vi "Lockin.Low Pass Filter (subVI).vi"(8 "error in (no error)":errorcluster, 9 "Element Data":i32, 10 "Array":waveform(dbl)[](array[waveform]), 11 "Lockin.DAQ in":refnum<class "Instrument.DAQ.lvclass">) -> (0 "error out":errorcluster, 1 "Fc (Hz)":dbl, 2 "signal out":waveform(dbl)[](array[waveform]))   [LabVIEW 2019, in "Instrument.DAQ.lvclass"]
uses:
  Instrument.DAQ.lvclass
  Instrument.DAQ.lvclass/Instrument.DAQ.ctl
  <vilib>/addons/Digital Filter Design/Process.llb/DFD Filtering (Array NChan).vi
  <vilib>/addons/Digital Filter Design/Process.llb/DFD Filtering (Wfm NChan).vi
  <vilib>/addons/Digital Filter Design/NI_DigFilterLicensed.lvlib
panel:
  out "Lockin.DAQ out":refnum<class "Instrument.DAQ.lvclass">
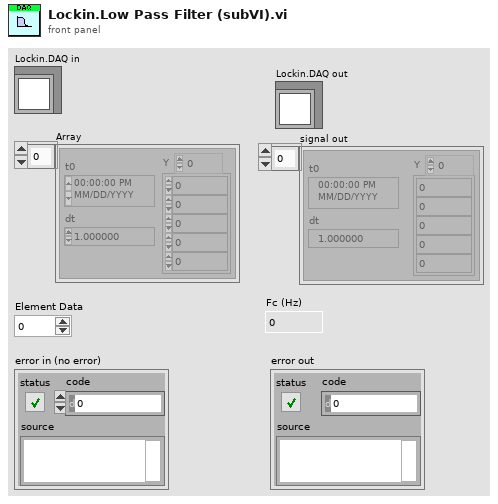
[diagram p1: front panel]
types:
  T1 = typedef "Instrument.DAQ.lvclass/REF.Channel--Cluster--Array.ctl" = T2[]
  T2 = typedef "Instrument.DAQ.lvclass/REF.Channel--Cluster.ctl" = cluster{"Enable?":bool, "Channel":i32, "Frequency":dbl, "Phase":dbl, "TC":dbl, "Roll-Off":i32}
  T3 = enum16{"Lowpass", "Highpass", "Bandpass", "Bandstop"}
  T4 = typedef "NI_DigFilterLicensed.lvlib/DFD Filter Obj.ctl" = cluster{"mSRate_Fs":dbl, "mSRate_Version":string, "mSRate_Comments":string, "mSRate_OrgCoef":T5, "mSRate_CurCoef":T5, "mSRate_Quantized?":bool, "mSRate_QCoef":T5, "mSRate_QSettings":T7[], "mSRate_Order":i32, "mSRate_Scaling":cluster{"mSRate_ScaleByPowerOf2?":bool, "mSRate_ScaleType":T9}}
  T5 = typedef "NI_DigFilterLicensed.lvlib/DFD Filter Coef.ctl" = cluster{"type":T6, "gain":dbl, "coef a (k)":dbl[], "coef b (v)":dbl[]}
  T6 = typedef "NI_DigFilterLicensed.lvlib/DFD Filter Structure Type Selector.ctl" = enum16{"Undefined", "FIR Direct Form", "FIR Direct Form Transposed", "FIR Symmetric", "FIR Antisymmetric", "IIR Direct Form I", "IIR Direct Form I Transposed", "IIR Direct Form II", "IIR Direct Form II Transposed", "IIR Cascaded Second Order Sections Form I", "IIR Cascaded Second Order Sections Form I Transposed", "IIR Cascaded Second Order Sections Form II", "IIR Cascaded Second Order Sections Form II Transposed", "Lattice Allpass (basic sections)", "Lattice Allpass (one multiplier sections)", "Lattice Allpass (normalized sections)", "Lattice AR (basic sections)", "Lattice AR (one multiplier sections)", "Lattice AR (normalized sections)", "Lattice MA (minimum phase)", "Lattice MA (maximum phase)", "Lattice ARMA (basic sections)", "Lattice ARMA (one multiplier sections)", "Lattice ARMA (normalized sections)"}
  T7 = typedef "NI_DigFilterLicensed.lvlib/dfd_Internal Quantization Settings.ctl" = cluster{"source":T8, "wl":i16, "iwl":i16, "overflow mode":enum16{"Saturation", "Wrap"}, "rounding mode":enum16{"Nearest", "Truncation"}, "signed?":bool}
  T8 = typedef "NI_DigFilterLicensed.lvlib/dfd_Internal Quantization Srcs.ctl" = u16
  T9 = typedef "NI_DigFilterLicensed.lvlib/DFD Coef Norm Type.ctl" = enum16{"No Norm", "Time Domain 1-Norm", "Time Domain 2-Norm", "Time Domain Inf-Norm"}
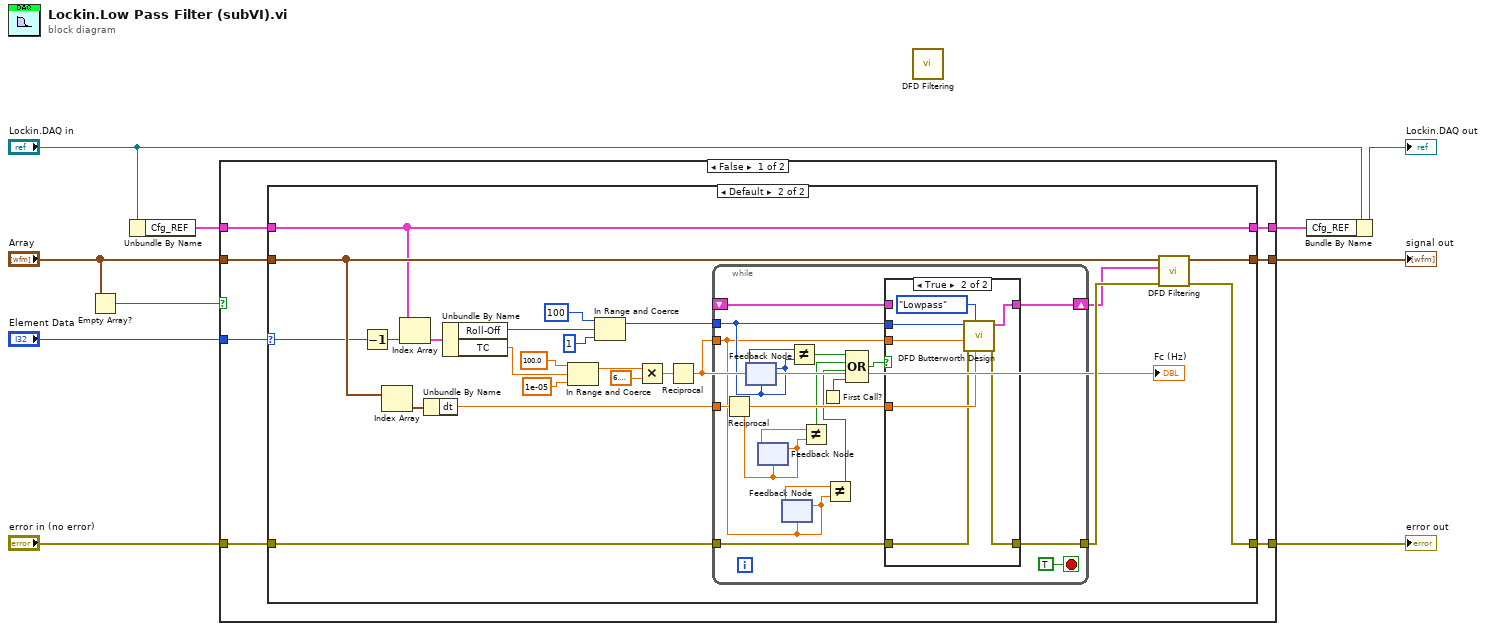
[diagram p0: block diagram]
diagram:
  n1 = Empty Array?(array="Array") -> (empty?=w6:bool)
  n2 = Unbundle By Name("Lockin.DAQ in") -> ("Cfg_REF"=w3:T1)
  n3 = case shown="False" w6 {
    tunnel: "error in (no error)" -> [w17 w72]
    tunnel: [w16 w72] -> w9
    tunnel: [w15 w71] -> w8
    tunnel: "Element Data" -> [w13 _]
    tunnel: "Array" -> [w14 w71]
    tunnel: w3 -> [w12 w70]
    tunnel: [w11 w70] -> w1
    frame False {
      n4 = case shown="Default" w13 {
        selector: w13 -> [_ w26]
        tunnel: w17 -> [w20 w43]
        tunnel: [w20 w22] -> w16
        tunnel: w14 -> [w19 w42]
        tunnel: [w19 w27] -> w15
        tunnel: w12 -> [w18 w21]
        tunnel: [w18 w21] -> w11
        frame 0 {
        }
        frame Default {
          n5 = Decrement(x=w26) -> (x-1=w25:i32)
          n6 = Index Array(array=w42) -> (element=w40:waveform(dbl))  [unwired: 1 in]
          n7 = Index Array(array=w21, index=w25) -> (element=w38:T2)
          n8 = Unbundle By Name(w40) -> ("dt"=w39:dbl)
          n9 = Unbundle By Name(w38) -> ("Roll-Off"=w36:i32, "TC"=w37:dbl)
          n10 = In Range and Coerce(upper limit=100.0, x=w37, lower limit=1e-05) -> (coerced(x)=w29:dbl)  [unwired: 1 out]
          n11 = In Range and Coerce(upper limit=100, x=w36, lower limit=1) -> (coerced(x)=w28:i32)  [unwired: 1 out]
          n12 = Multiply(x=w29, y=6.283185307179586) -> (x*y=w33:dbl)
          n13 = Reciprocal(x=w33) -> (1/x=w24:dbl)
          "Fc (Hz)" <- w24
          n14 = while {
            tunnel: w39 -> [w60]
            tunnel: w28 -> [w55]
            tunnel: w24 -> [w51]
            shift-right: [w46] -> w23
            shift-left: _ -> [w47]
            tunnel: w43 -> [w58]
            tunnel: [w57] -> w41
            stop <- TRUE stop-if-true
            n15 = Reciprocal(x=w60) -> (1/x=w53:dbl)
            n16 = feedback-in #1(w55) -> ()
            n17 = feedback #1(w55) -> (w56:i32)
            n18 = feedback #2(w53) -> (w54:dbl)
            n19 = feedback-in #2(w53) -> ()
            n20 = feedback #3(w51) -> (w52:dbl)
            n21 = feedback-in #3(w51) -> ()
            n22 = Not Equal?(x=w56, y=w55) -> (x != y?=w50:bool)
            n23 = Not Equal?(x=w54, y=w53) -> (x != y?=w49:bool)
            n24 = First Call?() -> (First Call?: T/F=w45:bool)
            n25 = Not Equal?(x=w52, y=w51) -> (x != y?=w48:bool)
            n26 = Compound Arithmetic op=OR(w50, w49, w48, w45) -> (w44:bool)
            n27 = case shown="True" w44 {
              tunnel: w53 -> [_ w69]
              tunnel: w55 -> [_ w67]
              tunnel: w51 -> [_ w66]
              tunnel: w58 -> [w62 w65]
              tunnel: [w62 w64] -> w57
              tunnel: [w61 w63] -> w46
              tunnel: w47 -> [w61 _]
              frame False {
              }
              frame True {
                n28 = call <vilib>:"DFD Butterworth Design.vi"("fs [Hz]"=w69, "filter type"=T3."Lowpass", "error in (no error)"=w65, "low cutoff freq [Hz]"=w66, "order"=w67) -> ("error out"=w64:errorcluster, "filter out"=w63:T4)  [unwired: 5 in]
              }
            }
          }
          n29 = call-poly <vilib>:"DFD Filtering.vi"("error in (no error)"=w41, "filter"=w23, "signal in"=w42) -> ("error out"=w22:errorcluster, "signal out"=w27:waveform(dbl)[])  [unwired: 7 in]
        }
      }
    }
    frame True {
    }
  }
  "error out" <- w9
  "signal out" <- w8
  n30 = call-poly <vilib>:"DFD Filtering.vi"() -> ()  [unwired: 10 in, 2 out]
  n31 = Bundle By Name(cluster="Lockin.DAQ in", "Cfg_REF"=w1) -> (→"Lockin.DAQ out":refnum<class "Instrument.DAQ.lvclass">)
